vi "Make wave_Cypher.vi"(10 "Totalpoints":dbl format="%#_6p") -> ()   [LabVIEW 2019]
doc: "This VI route the \"XMove\", \"YMove\" waves to two physical DAC channels in AFM."
panel:
  out "History":string="%fprintf 0, \"%f\",td_ReadValue(\"difference%laser\")\r"
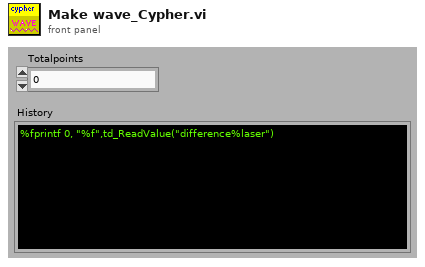
[diagram p1: front panel]
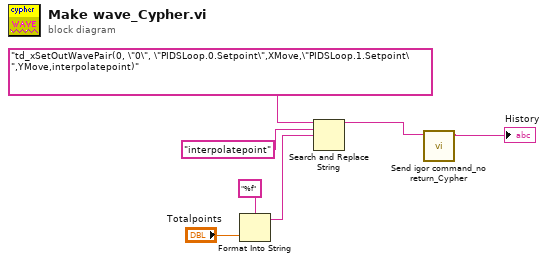
[diagram p0: block diagram]
diagram:
  n1 = Format Into String(format string="%f", "Totalpoints") -> (resulting string=w4:string)  [unwired: 2 in, 1 out]
  n2 = Search and Replace String(input string="td_xSetOutWavePair(0, \"0\", \"PIDSLoop.0.Setpoint\",XMove,\"PIDSLoop.1.Setpoint\",YMove,interpolatepoint)", search string="interpolatepoint", replace string=w4) -> (result string=w2:string)  [unwired: 1 in, 7 out]
  n3 = call "Send igor command_no return_Cypher.vi"("Command"=w2) -> ("History"=→"History":string)  [unwired: 10 out]
